vi "2D I64.vi"(5 "format string (%.;%#_20d)":string="%.;%#_20d", 7 "key description":string, 8 "sections":string[](array[string]), 9 "numeric":i64[][](array[numeric]), 11 "info data":string) -> (3 "info data out":string)   [LabVIEW 2020, in "infolib.lvlib"]
doc: "Add a new numeric table to Info Data string. If section exists in Info Data string, inserts key into this section."
uses:
  infolib.lvlib
panel:
  out "sections out":string[](array[string])
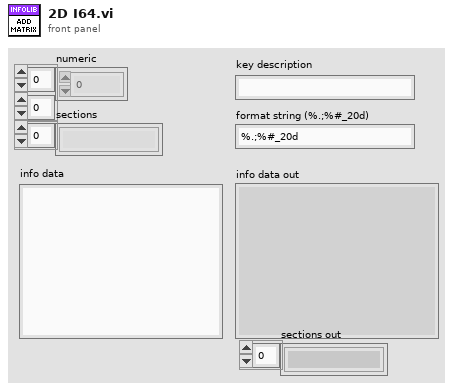
[diagram p1: front panel]
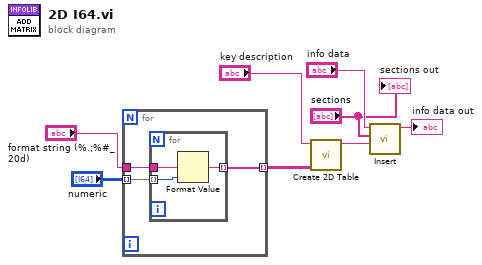
[diagram p0: block diagram]
diagram:
  n1 = for {
    tunnel: "format string (%.;%#_20d)" -> [w11]
    tunnel: "numeric" -> [w10] mode=indexing
    tunnel: [w9] -> w3 mode=indexing
    n2 = for {
      tunnel: w11 -> [w14]
      tunnel: w10 -> [w13] mode=indexing
      tunnel: [w12] -> w9 mode=indexing
      n3 = Format Value(format string=w14, value (0)=w13) -> (output string=w12:string)  [unwired: 1 in]
    }
  }
  n4 = call "Create 2D Table.vi"("formatted values"=w3, "table name"="key description") -> ("table"=w1:string)  [unwired: 8 in, 1 out]
  n5 = call "Insert.vi"("insert"=w1, "sections"="sections", "info data"="info data") -> ("info data out"=→"info data out":string)  [unwired: 8 in]
  "sections out" <- "sections"
